vi "Build Demo Config.vi"() -> ()   [LabVIEW 2020, in "CDM-Config.lvlib"]
uses:
  CDM-Config.lvlib
  Meta Data.ctl
  Config Manager/Config Manager.lvclass/Config Manager.ctl
  Config Element/Set Owner.vi
  Config Element/Config Element.lvclass
  Config Manager/Config Manager.lvclass
panel:
  in  "Tree":string(tree)
  out "error out":errorcluster
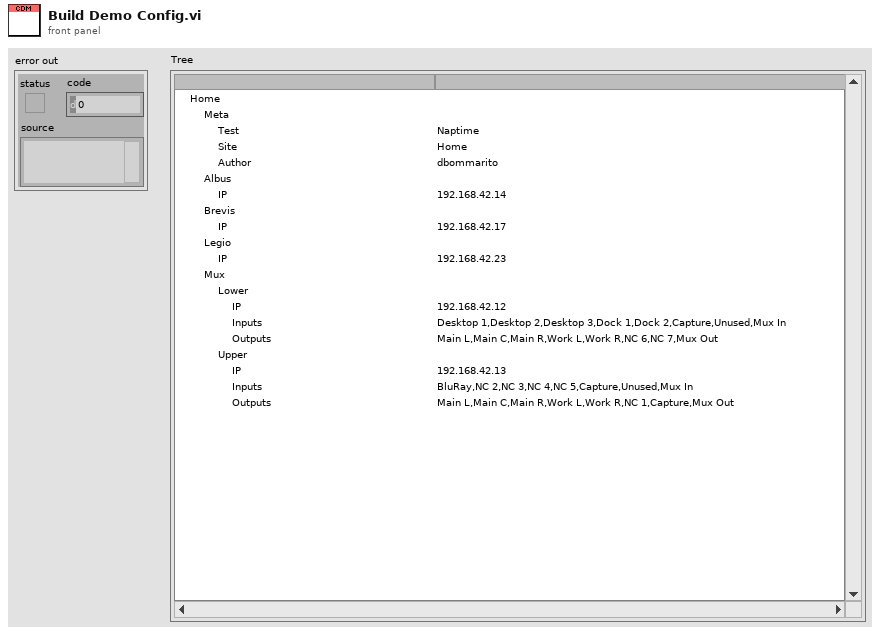
[diagram p1: front panel]
types:
  T1 = typedef "CDM-Config.lvlib/Meta Data.ctl" = cluster{"Name":string, "Value":string}
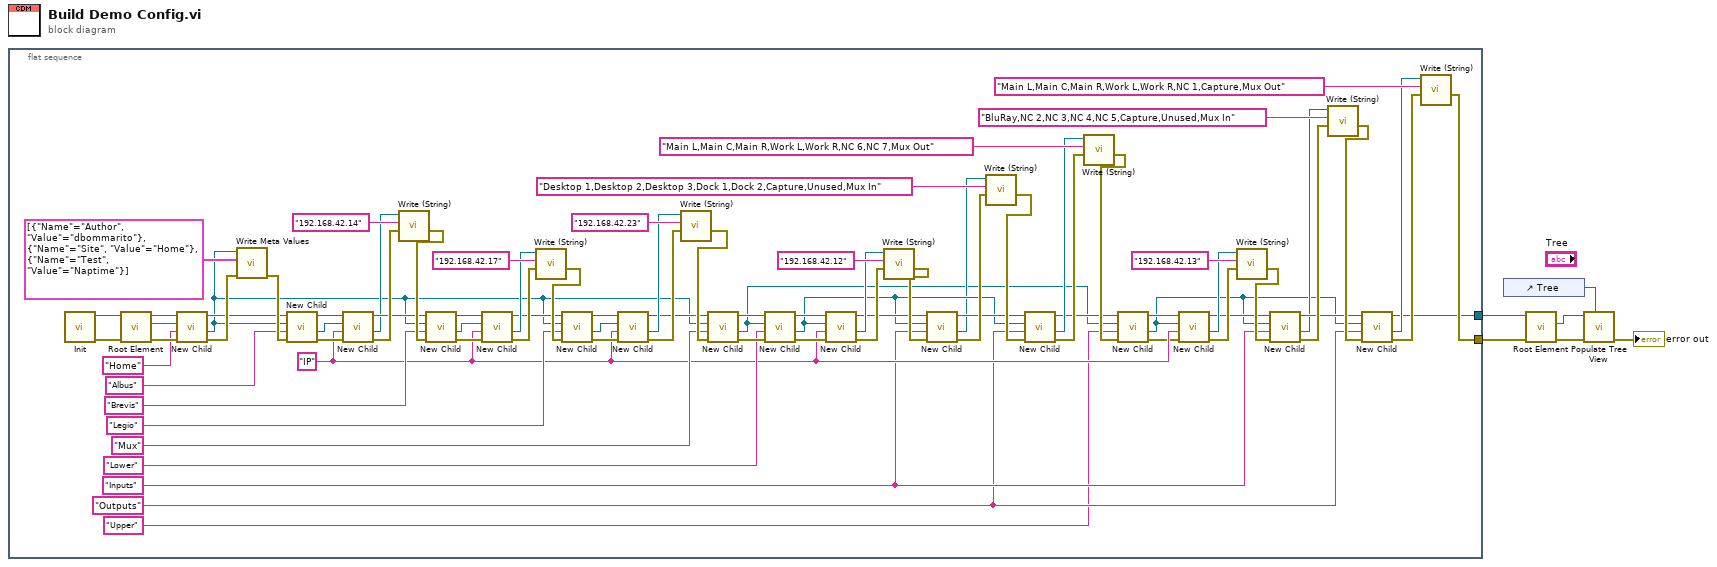
[diagram p0: block diagram]
diagram:
  n1 = flat-sequence {
    tunnel: [w8] -> w4
    tunnel: [w7] -> w3
    frame #0 {
      w18 = "Outputs" ("Child Name")
      w20 = "Inputs" ("Child Name")
      w24 = "IP" ("Child Name")
      n2 = call "Init.vi"() -> ("error out"=w65:errorcluster, "Config Manager out"=w70:refnum<class "Config Manager.lvclass">)  [unwired: 10 in]
      n3 = call "Root Element.vi"("error in (no error)"=w65, "Config Manager in"=w70) -> ("error out"=w68:errorcluster, "Root Element"=w67:refnum<class "Config Element.lvclass">, "Config Manager out"=w69:refnum<class "Config Manager.lvclass">)  [unwired: 7 in]
      n4 = call "New Child.vi"("error in (no error)"=w68, "Child Name"="Home", "Parent"=w67, "Config Manager in"=w69) -> ("error out"=w72:errorcluster, "New Child"=w42:refnum<class "Config Element.lvclass">, "Config Manager out"=w64:refnum<class "Config Manager.lvclass">)  [unwired: 5 in]
      n5 = call "Write Meta Values.vi"("error in (no error)"=w72, "Meta Data"=T1[] [{"Name"="Author", "Value"="dbommarito"}, {"Name"="Site", "Value"="Home"}, {"Name"="Test", "Value"="Naptime"}], "Config Element in"=w42) -> ("error out"=w73:errorcluster)  [unwired: 7 in, 1 out]
      n6 = call "New Child.vi"("error in (no error)"=w73, "Child Name"="Albus", "Parent"=w42, "Config Manager in"=w64) -> ("error out"=w60:errorcluster, "New Child"=w59:refnum<class "Config Element.lvclass">, "Config Manager out"=w61:refnum<class "Config Manager.lvclass">)  [unwired: 5 in]
      n7 = call "New Child.vi"("error in (no error)"=w60, "Child Name"=w24, "Parent"=w59, "Config Manager in"=w61) -> ("error out"=w89:errorcluster, "New Child"=w50:refnum<class "Config Element.lvclass">, "Config Manager out"=w57:refnum<class "Config Manager.lvclass">)  [unwired: 5 in]
      n8 = call "Write (String).vi"("error in (no error)"=w89, "String Value"="192.168.42.14", "Config Element in"=w50) -> ("error out"=w88:errorcluster)  [unwired: 7 in, 1 out]
      n9 = call "New Child.vi"("error in (no error)"=w88, "Child Name"="Brevis", "Parent"=w42, "Config Manager in"=w57) -> ("error out"=w54:errorcluster, "New Child"=w52:refnum<class "Config Element.lvclass">, "Config Manager out"=w55:refnum<class "Config Manager.lvclass">)  [unwired: 5 in]
      n10 = call "New Child.vi"("error in (no error)"=w54, "Child Name"=w24, "Parent"=w52, "Config Manager in"=w55) -> ("error out"=w87:errorcluster, "New Child"=w51:refnum<class "Config Element.lvclass">, "Config Manager out"=w48:refnum<class "Config Manager.lvclass">)  [unwired: 5 in]
      n11 = call "Write (String).vi"("error in (no error)"=w87, "String Value"="192.168.42.17", "Config Element in"=w51) -> ("error out"=w86:errorcluster)  [unwired: 7 in, 1 out]
      n12 = call "New Child.vi"("error in (no error)"=w86, "Child Name"="Legio", "Parent"=w42, "Config Manager in"=w48) -> ("error out"=w71:errorcluster, "New Child"=w46:refnum<class "Config Element.lvclass">, "Config Manager out"=w47:refnum<class "Config Manager.lvclass">)  [unwired: 5 in]
      n13 = call "New Child.vi"("error in (no error)"=w71, "Child Name"=w24, "Parent"=w46, "Config Manager in"=w47) -> ("error out"=w85:errorcluster, "New Child"=w44:refnum<class "Config Element.lvclass">, "Config Manager out"=w43:refnum<class "Config Manager.lvclass">)  [unwired: 5 in]
      n14 = call "Write (String).vi"("error in (no error)"=w85, "String Value"="192.168.42.23", "Config Element in"=w44) -> ("error out"=w84:errorcluster)  [unwired: 7 in, 1 out]
      n15 = call "New Child.vi"("error in (no error)"=w84, "Child Name"="Mux", "Parent"=w42, "Config Manager in"=w43) -> ("error out"=w39:errorcluster, "New Child"=w25:refnum<class "Config Element.lvclass">, "Config Manager out"=w40:refnum<class "Config Manager.lvclass">)  [unwired: 5 in]
      n16 = call "New Child.vi"("error in (no error)"=w39, "Child Name"="Lower", "Parent"=w25, "Config Manager in"=w40) -> ("error out"=w35:errorcluster, "New Child"=w31:refnum<class "Config Element.lvclass">, "Config Manager out"=w36:refnum<class "Config Manager.lvclass">)  [unwired: 5 in]
      n17 = call "New Child.vi"("error in (no error)"=w35, "Child Name"=w24, "Parent"=w31, "Config Manager in"=w36) -> ("error out"=w83:errorcluster, "New Child"=w34:refnum<class "Config Element.lvclass">, "Config Manager out"=w33:refnum<class "Config Manager.lvclass">)  [unwired: 5 in]
      n18 = call "Write (String).vi"("error in (no error)"=w83, "String Value"="192.168.42.12", "Config Element in"=w34) -> ("error out"=w82:errorcluster)  [unwired: 7 in, 1 out]
      n19 = call "New Child.vi"("error in (no error)"=w82, "Child Name"=w20, "Parent"=w31, "Config Manager in"=w33) -> ("error out"=w81:errorcluster, "New Child"=w29:refnum<class "Config Element.lvclass">, "Config Manager out"=w32:refnum<class "Config Manager.lvclass">)  [unwired: 5 in]
      n20 = call "Write (String).vi"("error in (no error)"=w81, "String Value"="Desktop 1,Desktop 2,Desktop 3,Dock 1,Dock 2,Capture,Unused,Mux In", "Config Element in"=w29) -> ("error out"=w80:errorcluster)  [unwired: 7 in, 1 out]
      n21 = call "New Child.vi"("error in (no error)"=w80, "Child Name"=w18, "Parent"=w31, "Config Manager in"=w32) -> ("error out"=w79:errorcluster, "New Child"=w27:refnum<class "Config Element.lvclass">, "Config Manager out"=w26:refnum<class "Config Manager.lvclass">)  [unwired: 5 in]
      n22 = call "Write (String).vi"("error in (no error)"=w79, "String Value"="Main L,Main C,Main R,Work L,Work R,NC 6,NC 7,Mux Out", "Config Element in"=w27) -> ("error out"=w78:errorcluster)  [unwired: 7 in, 1 out]
      n23 = call "New Child.vi"("error in (no error)"=w78, "Child Name"="Upper", "Parent"=w25, "Config Manager in"=w26) -> ("error out"=w12:errorcluster, "New Child"=w10:refnum<class "Config Element.lvclass">, "Config Manager out"=w11:refnum<class "Config Manager.lvclass">)  [unwired: 5 in]
      n24 = call "New Child.vi"("error in (no error)"=w12, "Child Name"=w24, "Parent"=w10, "Config Manager in"=w11) -> ("error out"=w77:errorcluster, "New Child"=w22:refnum<class "Config Element.lvclass">, "Config Manager out"=w21:refnum<class "Config Manager.lvclass">)  [unwired: 5 in]
      n25 = call "Write (String).vi"("error in (no error)"=w77, "String Value"="192.168.42.13", "Config Element in"=w22) -> ("error out"=w76:errorcluster)  [unwired: 7 in, 1 out]
      n26 = call "New Child.vi"("error in (no error)"=w76, "Child Name"=w20, "Parent"=w10, "Config Manager in"=w21) -> ("error out"=w75:errorcluster, "New Child"=w16:refnum<class "Config Element.lvclass">, "Config Manager out"=w19:refnum<class "Config Manager.lvclass">)  [unwired: 5 in]
      n27 = call "Write (String).vi"("error in (no error)"=w75, "String Value"="BluRay,NC 2,NC 3,NC 4,NC 5,Capture,Unused,Mux In", "Config Element in"=w16) -> ("error out"=w74:errorcluster)  [unwired: 7 in, 1 out]
      n28 = call "New Child.vi"("error in (no error)"=w74, "Child Name"=w18, "Parent"=w10, "Config Manager in"=w19) -> ("error out"=w9:errorcluster, "New Child"=w14:refnum<class "Config Element.lvclass">, "Config Manager out"=w7:refnum<class "Config Manager.lvclass">)  [unwired: 5 in]
      n29 = call "Write (String).vi"("error in (no error)"=w9, "String Value"="Main L,Main C,Main R,Work L,Work R,NC 1,Capture,Mux Out", "Config Element in"=w14) -> ("error out"=w8:errorcluster)  [unwired: 7 in, 1 out]
    }
  }
  n30 = control-ref of="Tree"() -> (w5:refnum<vi>)
  n31 = call "Root Element.vi"("error in (no error)"=w4, "Config Manager in"=w3) -> ("error out"=w2:errorcluster, "Root Element"=w1:refnum<class "Config Element.lvclass">)  [unwired: 7 in, 1 out]
  n32 = call "Populate Tree View.vi"("Tree"=w5, "error in (no error)"=w2, "Element"=w1) -> ("error out"=→"error out":errorcluster)  [unwired: 8 in]
